vi "TimeWizard.vi"(0 "Separator":string(combo), 1 "Weekday":string(combo), 3 "Hour":string(combo), 4 "Second":string(combo), 5 "Year":string(combo), 6 "AM/PM":string(combo), 9 "Month":string(combo), 10 "Search String":string, 11 "Day":string(combo), 12 "Time Zone":string(combo), 13 "Minute":string(combo), 15 "Select Time Zone":i32(listbox)) -> (2 "TZ Shift (sec)":dbl format="%#_6f", 8 "Format String":string, 14 "Formatted date/time string":string)   [LabVIEW 2015]
panel:
  out "Index Subset":i32[](array[numeric])
  in  "stop":bool
  out "Locale Time Stamp":timestamp=timestamp(3357626462.919444 s since 1904-01-01) format="%<%I:%M:%S %p\n%m/%d/%y>T"
  out "UTC Time Stamp":timestamp=timestamp(3357626462.919444 s since 1904-01-01) format="%<%I:%M:%S %p\n%m/%d/%y>T"
  # "Add formatting options so that user can adjust according to needs\nmaybe make displaying clock time an option\nhow should dd mmm yyyy be displayed, etc.\nthen pass those controls through this vi to produce the \"locale time stamp\" (presumably)"
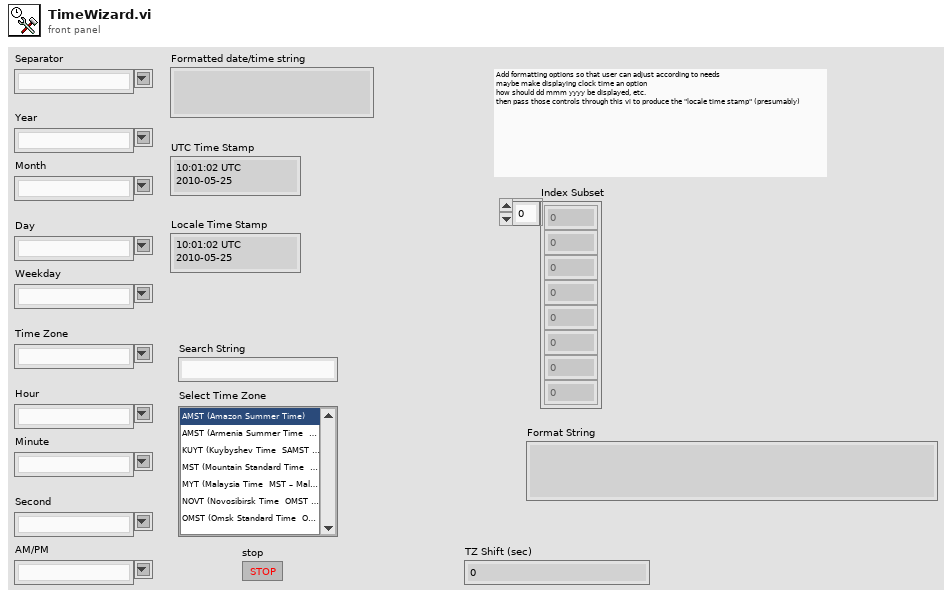
[diagram p1: front panel]
types:
  T1 = enum32{"Bad", "Idle", "Run top level", "Running"}
  T2 = typedef "LVDateTimeRec.ctl" = cluster{"fractional second":dbl, "second":i32, "minute":i32, "hour":i32, "day of month":i32, "month":i32, "year":i32, "day of week":i32, "day of year":i32, "DST":i32}
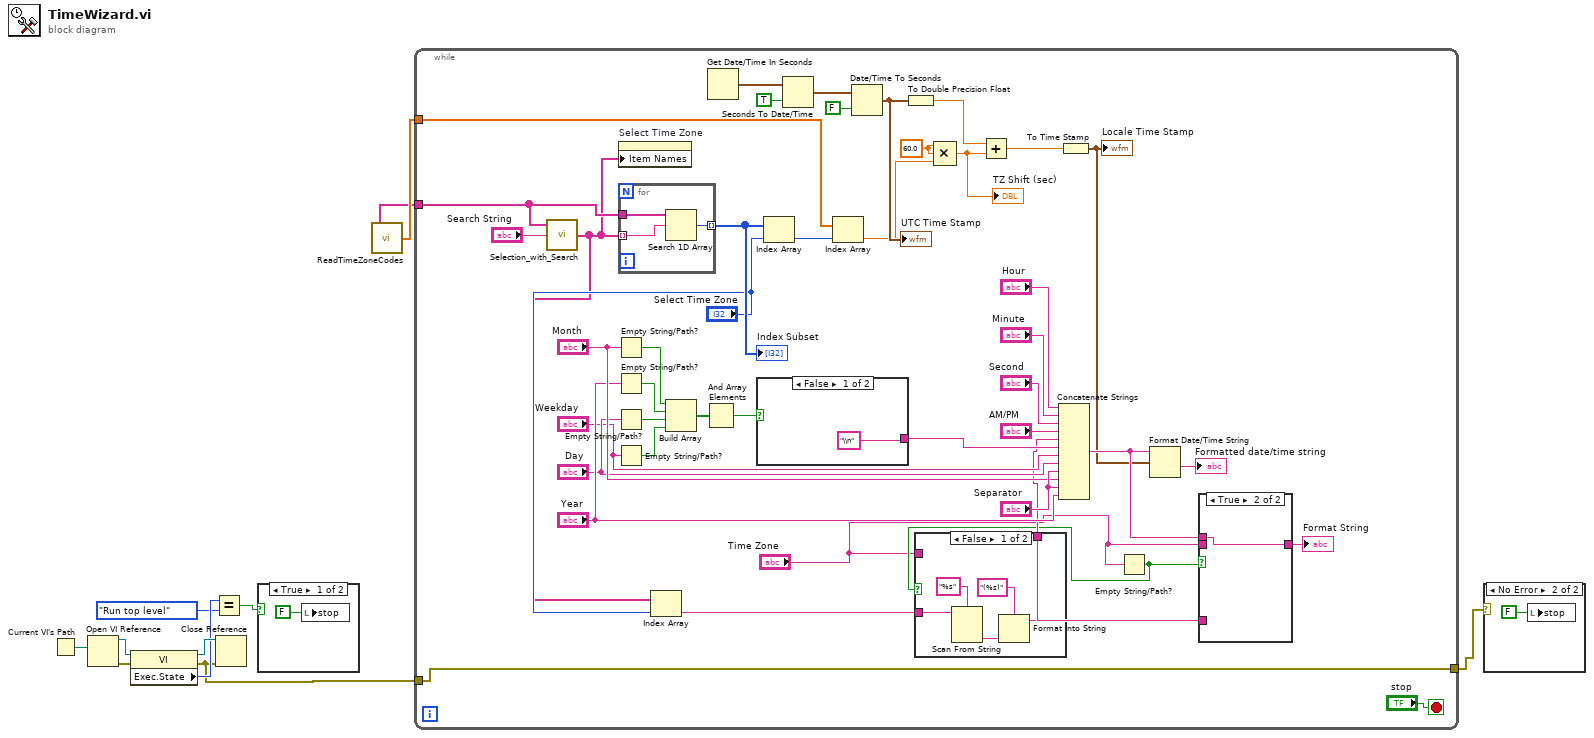
[diagram p0: block diagram]
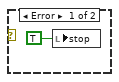
[diagram p2: hidden frame]
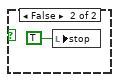
[diagram p3: hidden frame]
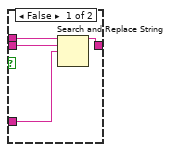
[diagram p5: hidden frame]
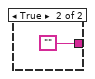
[diagram p6: hidden frame]
diagram:
  n1 = Current VI's Path() -> (path=w9:path)
  n2 = Open VI Reference(vi path=w9) -> (vi reference=w8:refnum<vi>, error out=w7:errorcluster)  [unwired: 5 in]
  n3 = property class="VI"(reference=w8, error in=w7) -> (reference out=w6:refnum<vi>, error out=w2:errorcluster, "Exec.State"=w5:T1)
  n4 = Equal?(x=w5, y=T1."Run top level" ("Execution:State 2")) -> (x = y?=w3:bool)
  n5 = Close Reference(reference=w6, error in (no error)=w2) -> ()  [unwired: 1 out]
  n6 = case shown="True" w3 {
    frame True {
      n7 = local write "stop"(FALSE) -> ()
    }
    frame False {
      n8 = local write "stop"(TRUE) -> ()
    }
  }
  n9 = call "ReadTimeZoneCodes.vi"() -> ("x+y"=w11:dbl[], "Abbreviation"=w10:string[])
  n10 = while {
    tunnel: w11 -> [w47]
    tunnel: w10 -> [w20]
    tunnel: w2 -> [w22]
    tunnel: [w22] -> w1
    stop <- "stop" stop-if-true
    w56 = 60.0 ("value")
    n11 = call "Selection_with_Search.vi"("Search String"="Search String", "All Channel Names"=w20) -> ("Item Names"=w17:string[])  [unwired: 1 in]
    n12 = Empty String/Path?(string/path="Month") -> (empty?=w31:bool)
    n13 = Empty String/Path?(string/path="Year") -> (empty?=w30:bool)
    n14 = Empty String/Path?(string/path="Day") -> (empty?=w29:bool)
    n15 = Empty String/Path?(string/path="Weekday") -> (empty?=w28:bool)
    n16 = property on="Select Time Zone" class="LstBox (strict)"("Item Names"=w17) -> ()  [unwired: 2 in, 2 out]
    n17 = for {
      tunnel: w20 -> [w72]
      tunnel: w17 -> [w71] mode=indexing
      tunnel: [w70] -> w44 mode=indexing
      n18 = Search 1D Array(1D array=w72, element=w71) -> (index of element=w70:i32)  [unwired: 1 in]
    }
    "Index Subset" <- w44
    n19 = Index Array(array=w17, index="Select Time Zone") -> (element=w18:string)
    n20 = Build Array(w31, w30, w29, w28) -> (w27:bool[])
    n21 = And Array Elements(Boolean array=w27) -> (logical AND=w26:bool)
    n22 = Get Date/Time In Seconds() -> (seconds since 1Jan1904=w49:timestamp)
    n23 = case shown="False" w26 {
      tunnel: ["\\n" ""] -> w36
      frame False {
      }
      frame True {
      }
    }
    n24 = Index Array(array=w44, index="Select Time Zone") -> (element=w43:i32)
    n25 = Seconds To Date/Time(time stamp (now)=w49, to UTC (F)=TRUE) -> (date time rec=w50:T2)
    n26 = Index Array(array=w47, index=w43) -> (element=w46:dbl)
    n27 = Date/Time To Seconds(1:FALSE ("is UTC (F)"), 2:w50) -> (0:w48:timestamp)
    "UTC Time Stamp" <- w48
    n28 = To Double Precision Float(number=w48) -> (double precision float=w55:dbl)
    n29 = Compound Arithmetic op=MULTIPLY(w56, w56, w46) -> (w21:dbl)
    "TZ Shift (sec)" <- w21
    n30 = Add(x=w55, y=w21) -> (x+y=w54:dbl)
    n31 = To Time Stamp(1:w54) -> (0:w23:timestamp)
    "Locale Time Stamp" <- w23
    n32 = Empty String/Path?(string/path="Time Zone") -> (empty?=w15:bool)
    n33 = case shown="False" w15 {
      tunnel: w18 -> [w60 _]
      tunnel: [w57 w62] -> w16
      tunnel: "Time Zone" -> [_ w62]
      frame False {
        n34 = Scan From String(format string="%s", input string=w60) -> (output 1=w59:string)  [unwired: 3 in, 3 out]
        n35 = Format Into String(format string="(%s)", w59) -> (resulting string=w57:string)  [unwired: 2 in, 1 out]
      }
      frame True {
      }
    }
    n36 = Concatenate Strings("Hour", "Minute", "Second", "AM/PM", w16, w36, "Weekday", "Day", "Separator", "Month", "Separator", "Year") -> (w25:string)
    n37 = Format Date/Time String(time format string (%c)=w25, seconds (now)=w23) -> (date/time string=→"Formatted date/time string":string)  [unwired: 1 in]
    n38 = case shown="True" w15 {
      tunnel: w25 -> [w66 w67]
      tunnel: [w65 w67] -> w24
      tunnel: "Time Zone" -> [w64 _]
      tunnel: w16 -> [w63 _]
      frame False {
        n39 = Search and Replace String(input string=w66, search string=w64, replace string=w63) -> (result string=w65:string)  [unwired: 5 in, 3 out]
      }
      frame True {
      }
    }
    "Format String" <- w24
  }
  n40 = case shown="No Error" w1 {
    frame Error {
      n41 = local write "stop"(TRUE) -> ()
    }
    frame No Error {
      n42 = local write "stop"(FALSE) -> ()
    }
  }
